vi "Read Measurement (Single Point).vi"(7 "Maximum Time (10000 ms)":i32=10000, 8 "error in (no error)":errorcluster, 9 "Data Type (0: Current)":i32(ring) items=["Current", "Status", "Time", "Charge", "Humidity", "Resistance", "Source", "Temperature", "Voltage"], 10 "Channel (1: Channel 1)":i32(ring)=1 items=["Channel 1"=1], 11 "VISA resource name":refnum<visa-resource-name>) -> (0 "error out":errorcluster, 2 "Measurement":dbl, 3 "VISA resource name out":refnum<visa-resource-name>)   [LabVIEW 2017, in "Keysight B2980 Series.lvlib"]
doc: "Initiate and fetch the latest data in series."
uses:
  Keysight B2980 Series.lvlib
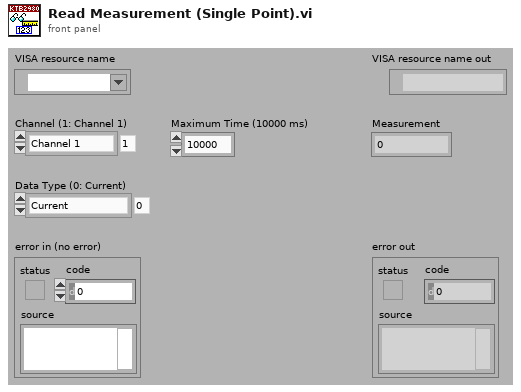
[diagram p1: front panel]
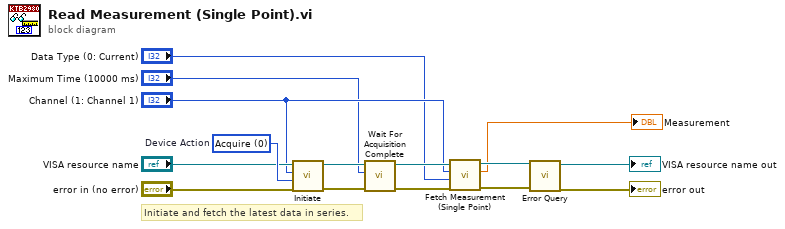
[diagram p0: block diagram]
diagram:
  w13 = 0 items=["Acquire", "Transient", "Both"]  # Device Action
  # "Initiate and fetch the latest data in series."
  n1 = call "Initiate.vi"("error in (no error)"="error in (no error)", "Device Action (2: Both)"=w13, "Channel (1: Channel 1)"="Channel (1: Channel 1)", "VISA resource name"="VISA resource name") -> ("error out"=w11:errorcluster, "VISA resource name out"=w12:refnum<visa-resource-name>)  [unwired: 6 out]
  n2 = call "Wait For Acquisition Complete.vi"("error in (no error)"=w11, "Maximum Time (10000 ms)"="Maximum Time (10000 ms)", "VISA resource name"=w12) -> ("error out"=w7:errorcluster, "VISA resource name out"=w8:refnum<visa-resource-name>)  [unwired: 7 out]
  n3 = call "Fetch Measurement (Single Point).vi"("error in (no error)"=w7, "Data Type (0: Current)"="Data Type (0: Current)", "Channel (1: Channel 1)"="Channel (1: Channel 1)", "VISA resource name"=w8) -> ("error out"=w5:errorcluster, "Measurement"=→"Measurement":dbl, "VISA resource name out"=w6:refnum<visa-resource-name>)  [unwired: 5 out]
  n4 = call "Error Query.vi"("error in (no error)"=w5, "VISA resource name"=w6) -> ("error out"=→"error out":errorcluster, "VISA resource name out"=→"VISA resource name out":refnum<visa-resource-name>)  [unwired: 8 out]
